vi "ExecuteCommand.vi"(10 "Params":string[][](array[string]), 11 "Command":string) -> ()   [LabVIEW 2017]
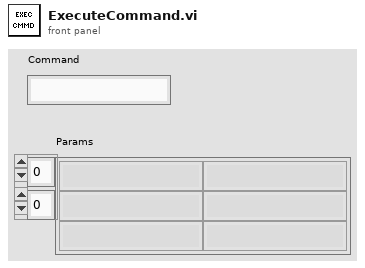
[diagram p1: front panel]
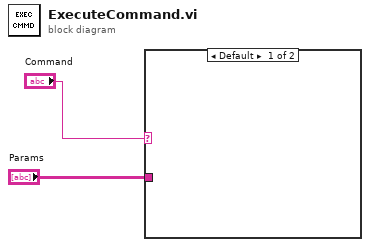
[diagram p0: block diagram]
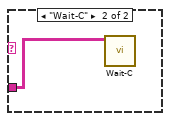
[diagram p2: hidden frame]
diagram:
  n1 = case shown="Default" "Command" {
    tunnel: "Params" -> [_ w3]
    frame Default {
    }
    frame "Wait-C" {
      n2 = call "Wait-C.vi"("Params"=w3) -> ()  [unwired: 11 in]
    }
  }
